vi "sub_trigger_vacuum_base.vi"(7 "cmd":enum16{"check", "clear"}(ring)) -> (3 "trigger":bool)   [LabVIEW 2013]
uses:
  ctl/UI_cmd-ctl.ctl
  <vilib>/Analysis/baseanly.llb/Mean (DBL).vi
  Global.vi
  <vilib>/Analysis/NI_AALBase.lvlib
panel:
  out "출력 클러스터":cluster{"Value":dbl, "force_cal":dbl}
  out "s? t:f":i32
  in  "count":i32=4
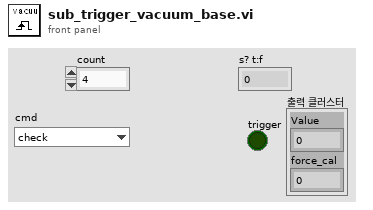
[diagram p1: front panel]
types:
  T1 = typedef "config_ctl.ctl" = cluster{"Trigger minlevel":dbl, "Lower Cut-Off":dbl, "Vacuum Trigger level":dbl, "state settings":cluster{"method":enum32{"histogram", "peak", "auto select"}, "histogram size":i32, "histogram method":enum16{"mode"}, "reserved":dbl}, "SPA-300 Setting":cluster{"Bonding force (g)":dbl, "Bonding time (ms)":dbl, "Pickup force (g)":dbl, "Pickup time (ms)":dbl, "Speed":enum16{"Slow", "Fast"}}}
  T2 = typedef "UI_cmd-ctl.ctl" = enum16{"default", "create", "read"}
  T3 = typedef "UI_ctl.ctl" = cluster{"Heater temp":refnum<vi>, "heater":refnum<vi>, "vacuum (kpa)":refnum<vi>, "Balance xy graph":refnum<vi>, "Strain chart w cal":refnum<vi>, "Pickup force":refnum<vi>, "Pickup time":refnum<vi>, "Data chart":refnum<vi>, "Trigger graph":refnum<vi>, "vacuum 차트":refnum<vi>, "vacuum":refnum<vi>, "Strain raw graph":refnum<vi>, "Strain raw chart":refnum<vi>, "Bonding time":refnum<vi>, "Bonding force":refnum<vi>, "Balance":refnum<vi>, "Filtered force graph":refnum<vi>, "ROI intensity":refnum<vi>, "Heater_rt":refnum<vi>, "Tensile force":refnum<vi>, "Force rt":refnum<vi>}
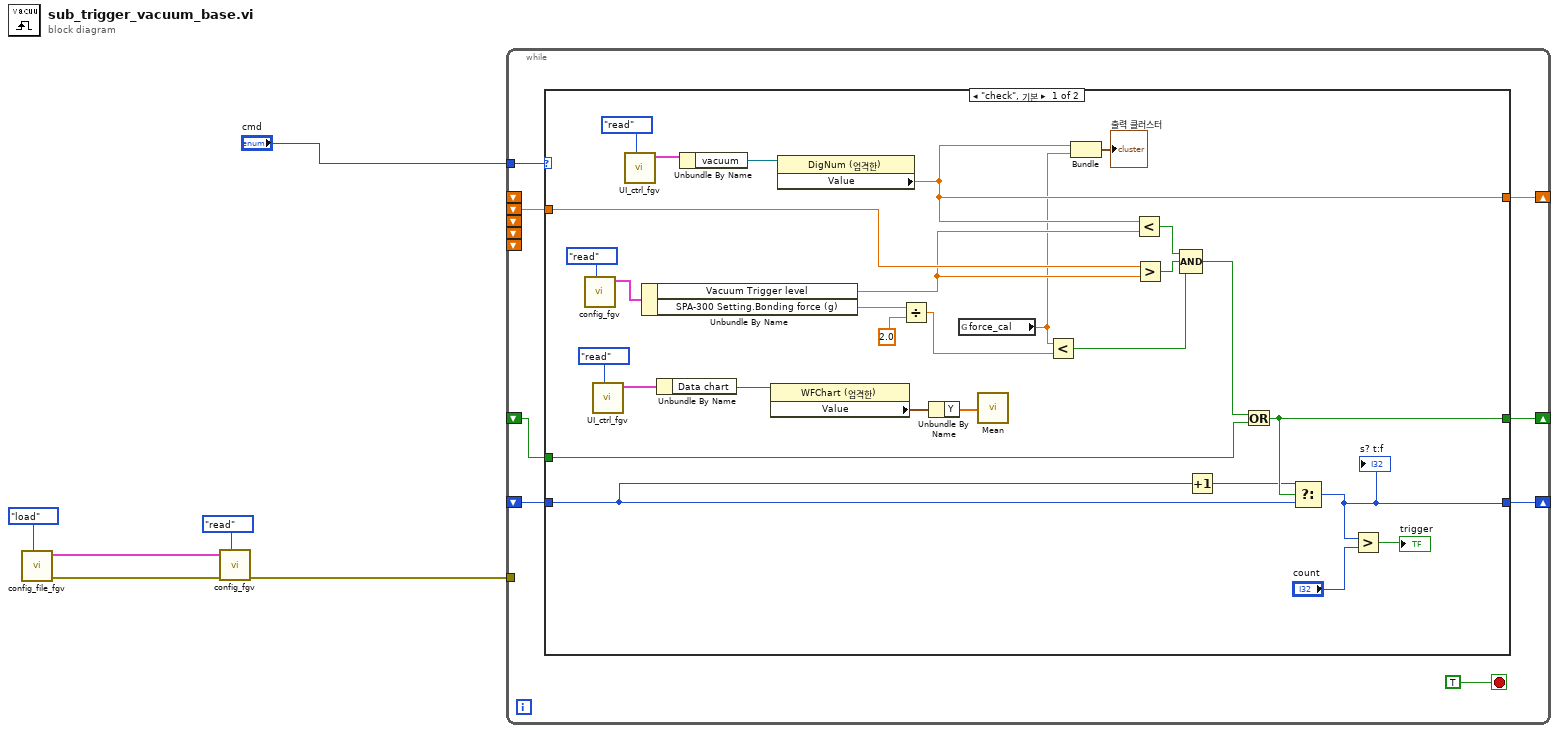
[diagram p0: block diagram]
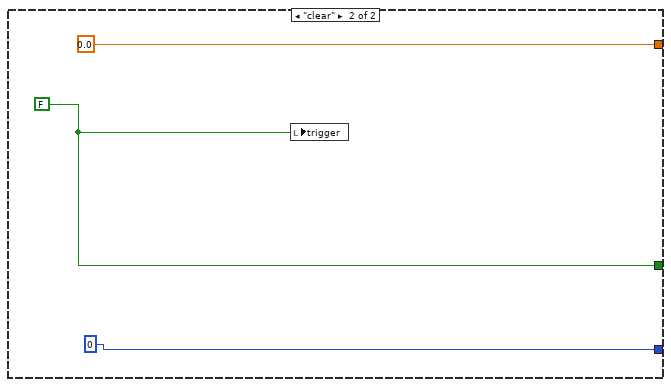
[diagram p2: hidden frame]
diagram:
  n1 = call "config_file_fgv.vi"("cmd"=enum16{"save", "load"}."load") -> ("error out"=w1:errorcluster, "var"=w2:T1)  [unwired: 8 in, 1 out]
  n2 = call "config_fgv.vi"("cmd"=enum16{"write", "read", "ini"}."read", "error in (no error)"=w1, "Config in"=w2) -> ("error out"=w4:errorcluster)  [unwired: 7 in, 1 out]
  n3 = while {
    tunnel: "cmd" -> [w13]
    shift-right: [w12] -> _
    shift-left: _ -> [_]
    shift-left: _ -> [w7]
    shift-left: _ -> [_]
    shift-left: _ -> [_]
    shift-left: _ -> [_]
    tunnel: w4 -> [_]
    shift-right: [w11] -> _
    shift-left: _ -> [w8]
    shift-right: [w10] -> _
    shift-left: _ -> [w9]
    stop <- TRUE stop-if-true
    n4 = case shown="\"check\", 기본" w13 {
      tunnel: [w17 0.0] -> w12
      tunnel: [w32 0] -> w11
      tunnel: [w36 w44] -> w10
      tunnel: w9 -> [w37 _]
      tunnel: w8 -> [w34 _]
      tunnel: w7 -> [w30 _]
      frame "check", Default {
        n5 = call "config_fgv.vi"("cmd"=enum16{"write", "read", "ini"}."read") -> ("Config out"=w28:T1)  [unwired: 9 in, 1 out]
        n6 = call "UI_ctrl_fgv.vi"("cmd"=UI_cmd-ctl."read") -> ("UI cluster out"=w23:T3)  [unwired: 10 in]
        n7 = call "UI_ctrl_fgv.vi"("cmd"=UI_cmd-ctl."read") -> ("UI cluster out"=w42:T3)  [unwired: 10 in]
        n8 = Unbundle By Name(w28) -> ("Vacuum Trigger level"=w27:dbl, "SPA-300 Setting.Bonding force (g)"=w25:dbl)
        n9 = Unbundle By Name(w23) -> ("Data chart"=w22:refnum<vi>)
        n10 = Unbundle By Name(w42) -> ("vacuum"=w41:refnum<vi>)
        n11 = property class="WFChart (엄격한)"(reference=w22) -> ("Value"=w21:waveform(dbl))  [unwired: 1 in, 2 out]
        n12 = property class="DigNum (엄격한)"(reference=w41) -> ("Value"=w17:dbl)  [unwired: 1 in, 2 out]
        n13 = Divide(x=w25, y=2.0) -> (x/y=w18:dbl)
        n14 = Unbundle By Name(w21) -> ("Y"=w20:dbl[])
        n15 = global read "Global.vi" "force_cal"() -> (w16:dbl)
        n16 = call-poly <vilib>:"Mean.vi"("X"=w20) -> ()  [unwired: 2 out]
        n17 = Less?(x=w16, y=w18) -> (x < y?=w19:bool)
        n18 = Bundle("Value"=w17, "force_cal"=w16) -> (→"출력 클러스터":cluster{"Value":dbl, "force_cal":dbl})  [unwired: 1 in]
        n19 = Less?(x=w17, y=w27) -> (x < y?=w39:bool)
        n20 = Greater?(x=w30, y=w27) -> (0:w40:bool)
        n21 = Compound Arithmetic op=AND(w39, w40, w19) -> (w38:bool)
        n22 = Increment(x=w34) -> (x+1=w35:i32)
        n23 = Or(x=w38, y=w37) -> (x .or. y?=w36:bool)
        n24 = Select(t=w35, s=w36, f=w34) -> (s? t:f=w32:i32)
        "s? t:f" <- w32
        n25 = Greater?(x=w32, y="count") -> (0:→"trigger":bool)
      }
      frame "clear" {
        w44 = FALSE
        n26 = local write "trigger"(w44) -> ()
      }
    }
  }
